vi "mqttCmdSend.vi"(0 "mqttBrokerCommand in":refnum<class "mqttCmd.lvclass">, 5 "byte1":u8, 11 "error in (no error)":errorcluster) -> (4 "mqttBrokerCommand out":refnum<class "mqttCmd.lvclass">, 15 "error out":errorcluster)   [LabVIEW 2020, in "mqttCmd.lvclass"]
uses:
  mqttCmd.lvclass
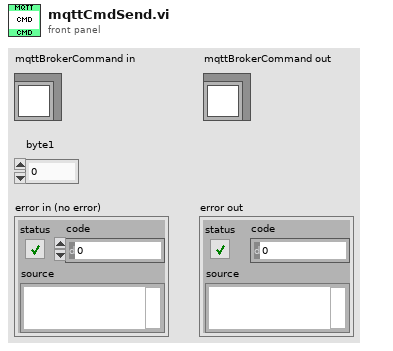
[diagram p1: front panel]
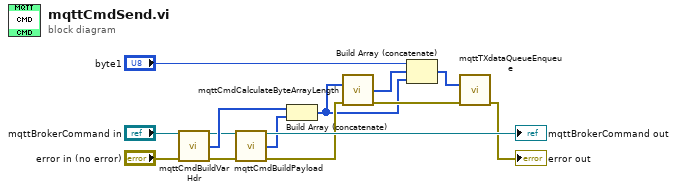
[diagram p0: block diagram]
diagram:
  n1 = call-dynamic "mqttCmdBuildVarHdr.vi"("_mqtt in"="mqttBrokerCommand in", "error in (no error)"="error in (no error)") -> ("_mqtt out"=w1:refnum<class "mqttCmd.lvclass">, "variableHeader"=w8:u8[], "error out"=w2:errorcluster)  [unwired: 11 in]
  n2 = call-dynamic "mqttCmdBuildPayload.vi"("_mqtt in"=w1, "error in (no error)"=w2) -> ("_mqtt out"=→"mqttBrokerCommand out":refnum<class "mqttCmd.lvclass">, "payload"=w9:u8[], "error out"=w7:errorcluster)  [unwired: 11 in]
  n3 = Build Array (concatenate)(w8, w9) -> (w6:u8[])
  n4 = call "mqttCmdCalculateByteArrayLength.vi"("byteArry in"=w6, "error in (no error)"=w7) -> ("length out"=w5:u8[], "error out"=w10:errorcluster)  [unwired: 12 in]
  n5 = Build Array (concatenate)("byte1", w5, w6) -> (w11:u8[])
  n6 = call "mqttTXdataQueueEnqueue.vi"("data in"=w11, "error in (no error)"=w10) -> ("error out"=→"error out":errorcluster)  [unwired: 13 in]
